vi "Test Calculate Curved Motion.vi"() -> ()   [LabVIEW 2024]
uses:
  <vilib>/Native 3D Graph/xcontrol/3DPC_SurfacePlot.xctl
  Vec3d Class/Vec3d.lvclass
panel:
  out "error out":errorcluster
  out "XY Graph":cluster{"X":dbl, "Y":dbl}[](graph)
  out "3D Graph":refnum<class "Base Datatype.lvclass">[](xcontrol)
  in  "orientation":enum16{"cw", "ccw"}(ring)
  in  "Points per revolution":u32=100
  in  "Speed (mm/s)":dbl
  in  "Radius":dbl
  in  "Destination XYZ":dbl[](array[numeric])
  in  "Origin XYZ":dbl[](array[numeric])
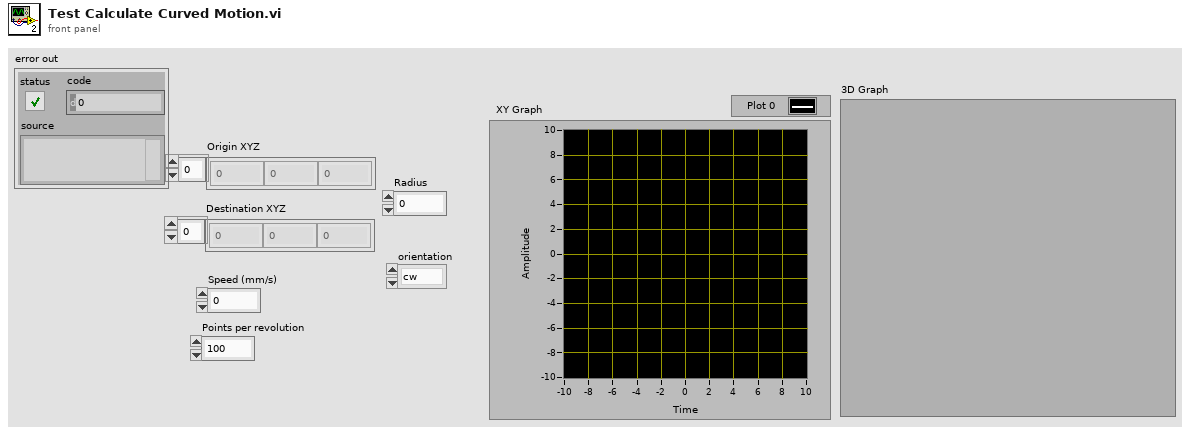
[diagram p1: front panel]
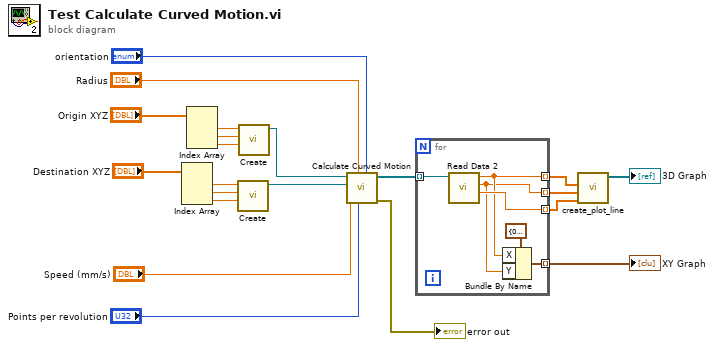
[diagram p0: block diagram]
diagram:
  n1 = Index Array(array="Destination XYZ") -> (element #1=w16:dbl, element #2=w15:dbl, element #3=w14:dbl)  [unwired: 3 in]
  n2 = Index Array(array="Origin XYZ") -> (element #1=w19:dbl, element #2=w18:dbl, element #3=w17:dbl)  [unwired: 3 in]
  n3 = call "Create.vi"("Z"=w14, "Y"=w15, "X"=w16) -> ("Vec3d Class out"=w12:refnum<class "Vec3d.lvclass">)  [unwired: 7 in, 1 out]
  n4 = call "Create.vi"("Z"=w17, "Y"=w18, "X"=w19) -> ("Vec3d Class out"=w13:refnum<class "Vec3d.lvclass">)  [unwired: 7 in, 1 out]
  n5 = call "Calculate Curved Motion.vi"("orientation"="orientation", "Points per revolution"="Points per revolution", "Radius"="Radius", "Speed (mm/s)"="Speed (mm/s)", "Destination"=w12, "Origin"=w13) -> ("error out"=→"error out":errorcluster, "Coordinates"=w6:refnum<class "Vec3d.lvclass">[])  [unwired: 2 in, 2 out]
  n6 = for {
    tunnel: w6 -> [w27] mode=indexing
    tunnel: [w24] -> w5 mode=indexing
    tunnel: [w23] -> w4 mode=indexing
    tunnel: [w26] -> w3 mode=indexing
    tunnel: [w22] -> w2 mode=indexing
    n7 = call-dynamic "Read Data 2.vi"("Vec3d in"=w27) -> ("Z"=w26:dbl, "Y"=w23:dbl, "X"=w24:dbl)  [unwired: 7 in, 1 out]
    n8 = Bundle By Name(cluster=cluster{"X":dbl, "Y":dbl} {"X"=0.0, "Y"=0.0}, "X"=w24, "Y"=w23) -> (w22:cluster{"X":dbl, "Y":dbl})
  }
  "XY Graph" <- w2
  n9 = call <vilib>:"create_plot_line.vi"("z vector"=w3, "y vector"=w4, "x vector"=w5) -> ("plots out"=→"3D Graph":refnum<class "Base Datatype.lvclass">[])  [unwired: 2 in, 6 out]
